vi "Write Step Config.lvclass.vi"(8 "error in (no error)":errorcluster, 10 "Step Config.lvclass":refnum<class "Step Config.lvclass">, 11 "StepNode in":refnum<class "StepNode.lvclass">) -> (0 "error out":errorcluster, 3 "StepNode out":refnum<class "StepNode.lvclass">)   [LabVIEW 2015, in "StepNode.lvclass"]
uses:
  StepNode.lvclass
  Prototype/classes/Step/Config/Step Config.lvclass
  StepNode.lvclass/StepNode.ctl
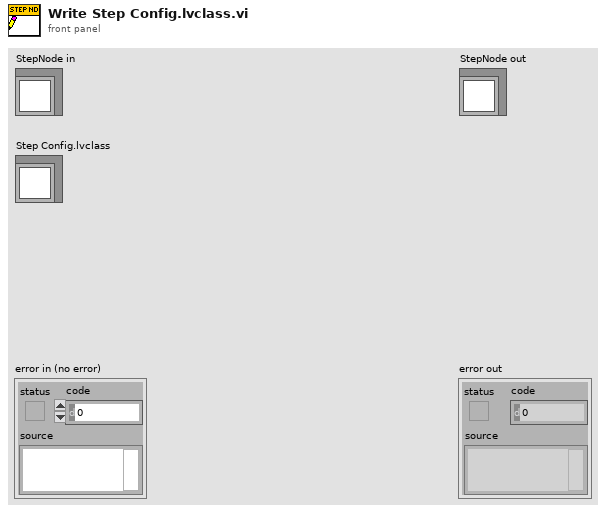
[diagram p1: front panel]
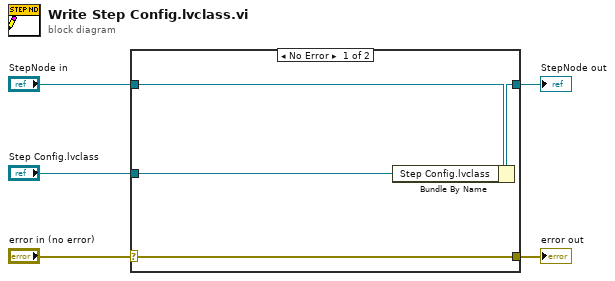
[diagram p0: block diagram]
diagram:
  n1 = case shown="No Error" "error in (no error)" {
    selector: "error in (no error)" -> [w9 w10]
    tunnel: [w9 w10] -> w4
    tunnel: [w7 w11] -> w2
    tunnel: "StepNode in" -> [w8 w11]
    tunnel: "Step Config.lvclass" -> [w6 _]
    frame No Error {
      n2 = Bundle By Name(cluster=w8, "Step Config.lvclass"=w6) -> (w7:refnum<class "StepNode.lvclass">)
    }
    frame Error {
    }
  }
  "error out" <- w4
  "StepNode out" <- w2
